vi "ensure_entry.vi"(9 "not found?":bool, 10 "id":string, 11 "named entries in":refnum<data-value>) -> (3 "named entries out":refnum<data-value>)   [LabVIEW 2019, in "Lookup API.lvlib" / "Mapped Lookup.lvclass"]
uses:
  Mapped Lookup.lvclass
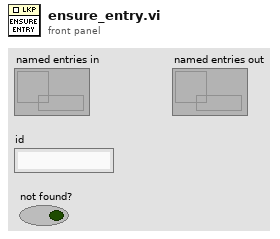
[diagram p1: front panel]
types:
  T1 = cluster{"instances":refnum<data-value>, "events":refnum<data-value>}
  T2 = map{string, cluster{"instances":refnum<data-value>, "events":refnum<data-value>}}
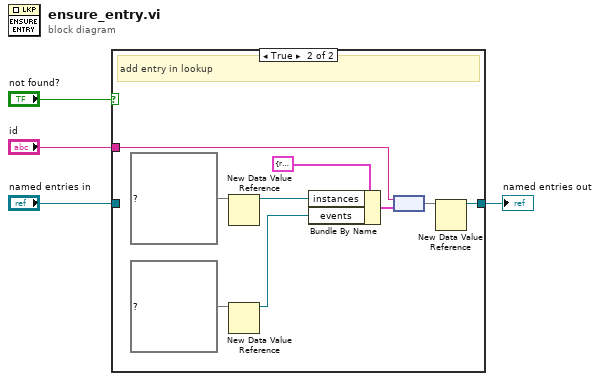
[diagram p0: block diagram]
diagram:
  n1 = case shown="True" "not found?" {
    tunnel: "named entries in" -> [w5 _]
    tunnel: [w5 w6] -> w3
    tunnel: "id" -> [_ w9]
    frame False {
    }
    frame True {
      # "add entry in lookup"
      n2 = New Data Value Reference(data value=set{refnum<data-value>} {}) -> (data value reference=w13:refnum<data-value>)  [unwired: 1 in, 1 out]
      n3 = New Data Value Reference(data value=set{refnum<user-event>} {}) -> (data value reference=w10:refnum<data-value>)  [unwired: 1 in, 1 out]
      n4 = Bundle By Name(cluster=T1 {"instances"=refnum, "events"=refnum}, "instances"=w13, "events"=w10) -> (w8:T1)
      n5 = node(w9, w8) -> (w7:T2)
      n6 = New Data Value Reference(data value=w7) -> (data value reference=w6:refnum<data-value>)  [unwired: 1 in, 1 out]
    }
  }
  "named entries out" <- w3
